vi "Actor Core.vi"(8 "error in":errorcluster, 11 "Nested in":refnum<class "Serial Devices.lvclass">) -> (0 "error out":errorcluster, 3 "Actor out":refnum<class "Actor.lvclass">)   [LabVIEW 2019, in "Serial Devices.lvlib" / "Serial Devices.lvclass"]
doc: "(<B>Filename</B>: Actor Framework.lvlib:Actor.lvclass:Actor Core.vi)\n\nReceives messages to the actor, reacts to them, and initiates any error handling that may shut the actor down.\n\nDescendant classes may override this VI to append parallel tasks for the actor to complete while it handles messages. Overrides use the Call Parent Method node."
uses:
  Serial Devices.lvclass
  <vilib>/ActorFramework/Actor/Actor.lvclass
  <vilib>/ActorFramework/Stop Msg/Stop Msg.lvclass
  Serial Devices Messages/AD Msg/AD Msg.lvclass
  C:/Program Files (x86)/National Instruments/LabVIEW 2019/vi.lib/ActorFramework/Actor/Actor.lvclass
panel:
  in  "Mandar Comando":bool
  in  "Pin":u8
  in  "Valor":u8
  in  "Puerto":u8
  in  "Canal":u8
  in  "Comandos":string(combo)="AD"
  out "Datos":string
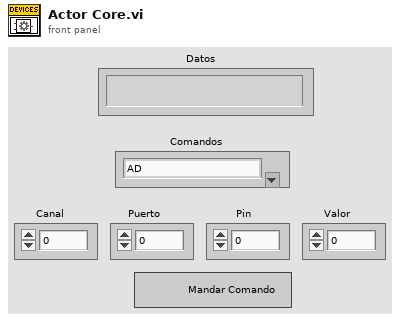
[diagram p1: front panel]
types:
  T1 = cluster{"Stop":refnum<user-event>, "Datos":refnum<user-event>}
  T2 = enum8{"Enabled", "Disabled", "Disabled and Grayed Out"}
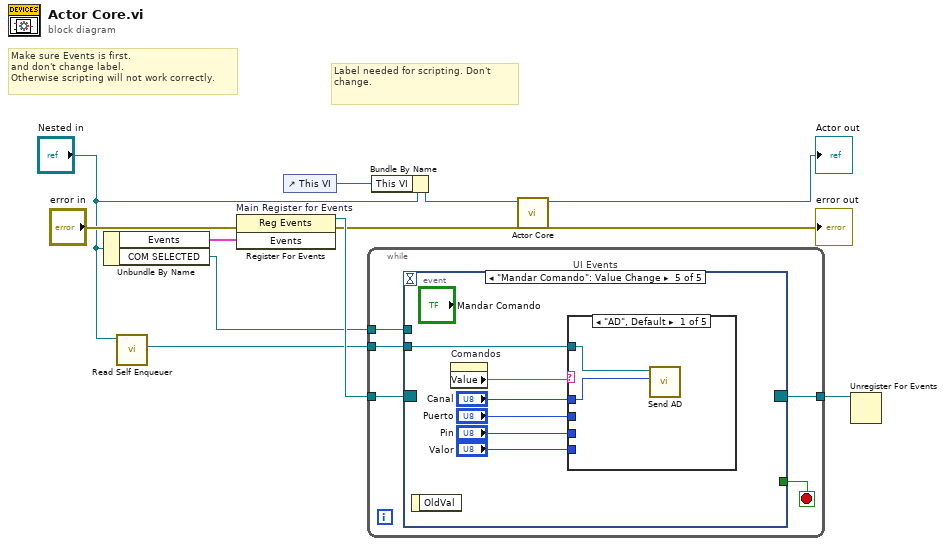
[diagram p0: block diagram]
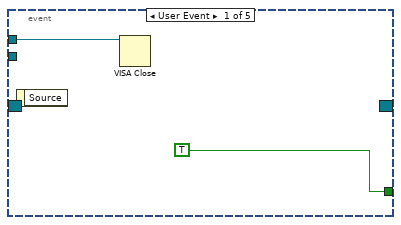
[diagram p2: hidden frame]
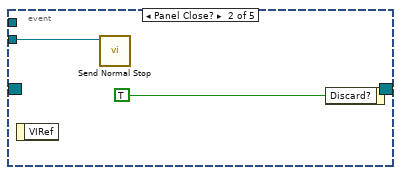
[diagram p3: hidden frame]
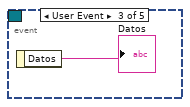
[diagram p4: hidden frame]
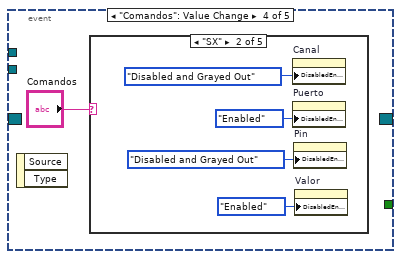
[diagram p5: hidden frame]
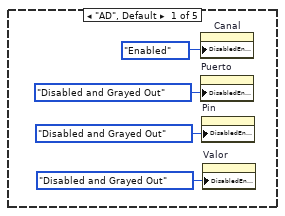
[diagram p6: hidden frame]
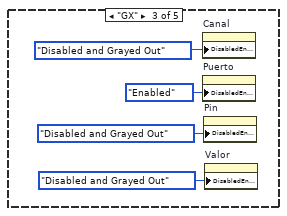
[diagram p7: hidden frame]
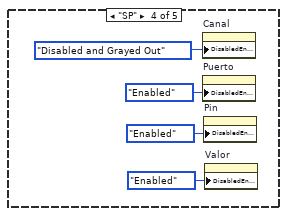
[diagram p8: hidden frame]
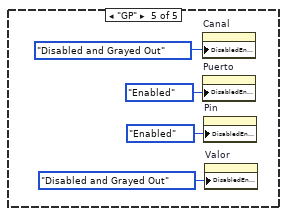
[diagram p9: hidden frame]
diagram:
  # "Label needed for scripting. Don't change."
  # "Make sure Events is first.\nand don't change label.\nOtherwise scripting will not work correctly."
  n1 = Unbundle By Name("Nested in") -> ("Events"=w9:T1, "COM SELECTED"=w1:refnum<visa-resource-name>)
  n2 = call <vilib>:"Read Self Enqueuer.vi"("Actor"="Nested in") -> ("Self Enqueuer"=w7:refnum<class "Message Enqueuer.lvclass">)  [unwired: 10 in]
  n3 = register-events "Main Register for Events"(error in="error in", w9) -> (reference out=w10:refnum<event-registration>, error out=w5:errorcluster)  [unwired: 1 in]
  n4 = control-ref of="This VI"() -> (w3:refnum<vi>)
  n5 = while {
    tunnel: w10 -> [w17]
    tunnel: [w15] -> w8
    tunnel: w7 -> [w14]
    tunnel: w1 -> [w13]
    stop <- w16 stop-if-true
    n6 = event "UI Events" shown="[4] \"Mandar Comando\": Value Change" {
      selector: w17 -> [_ _ _ _ _]
      dyn-events: [_ _ _ _ _] -> w15
      timeout: _ -> [_ _ _ _ _]
      tunnel: [TRUE _ _ _ _] -> w16
      tunnel: w14 -> [_ w20 _ _ w44]
      tunnel: w13 -> [w18 _ _ _ _]
      event User Event {
        n7 = event-data() -> ()  [unwired: 1 in, 1 out]
        n8 = VISA Close(VISA resource name=w18) -> ()  [unwired: 1 in, 1 out]
      }
      event Panel Close? {
        n9 = event-data() -> ()  [unwired: 1 in, 1 out]
        n10 = call <vilib>:"Send Normal Stop.vi"("Message Enqueuer"=w20) -> ()  [unwired: 10 in, 1 out]
        n11 = event-data("Discard?"=TRUE) -> ()  [unwired: 1 in, 1 out]
      }
      event User Event {
        n12 = event-data() -> ("Datos"=→"Datos":string)  [unwired: 1 in]
      }
      event "Comandos": Value Change {
        n13 = event-data() -> ()  [unwired: 1 in, 2 out]
        n14 = case shown="\"SX\"" "Comandos" {
          frame "AD", Default {
            n15 = property on="Canal" class="DigNum (strict)"("DisabledEnum"=T2."Enabled" ("Disabled")) -> ()  [unwired: 2 in, 2 out]
            n16 = property on="Puerto" class="DigNum (strict)"("DisabledEnum"=T2."Disabled and Grayed Out" ("Disabled")) -> ()  [unwired: 2 in, 2 out]
            n17 = property on="Pin" class="DigNum (strict)"("DisabledEnum"=T2."Disabled and Grayed Out" ("Disabled")) -> ()  [unwired: 2 in, 2 out]
            n18 = property on="Valor" class="DigNum (strict)"("DisabledEnum"=T2."Disabled and Grayed Out" ("Disabled")) -> ()  [unwired: 2 in, 2 out]
          }
          frame "SX" {
            n19 = property on="Canal" class="DigNum (strict)"("DisabledEnum"=T2."Disabled and Grayed Out" ("Disabled")) -> ()  [unwired: 2 in, 2 out]
            n20 = property on="Puerto" class="DigNum (strict)"("DisabledEnum"=T2."Enabled" ("Disabled")) -> ()  [unwired: 2 in, 2 out]
            n21 = property on="Pin" class="DigNum (strict)"("DisabledEnum"=T2."Disabled and Grayed Out" ("Disabled")) -> ()  [unwired: 2 in, 2 out]
            n22 = property on="Valor" class="DigNum (strict)"("DisabledEnum"=T2."Enabled" ("Disabled")) -> ()  [unwired: 2 in, 2 out]
          }
          frame "GX" {
            n23 = property on="Canal" class="DigNum (strict)"("DisabledEnum"=T2."Disabled and Grayed Out" ("Disabled")) -> ()  [unwired: 2 in, 2 out]
            n24 = property on="Puerto" class="DigNum (strict)"("DisabledEnum"=T2."Enabled" ("Disabled")) -> ()  [unwired: 2 in, 2 out]
            n25 = property on="Pin" class="DigNum (strict)"("DisabledEnum"=T2."Disabled and Grayed Out" ("Disabled")) -> ()  [unwired: 2 in, 2 out]
            n26 = property on="Valor" class="DigNum (strict)"("DisabledEnum"=T2."Disabled and Grayed Out" ("Disabled")) -> ()  [unwired: 2 in, 2 out]
          }
          frame "SP" {
            n27 = property on="Canal" class="DigNum (strict)"("DisabledEnum"=T2."Disabled and Grayed Out" ("Disabled")) -> ()  [unwired: 2 in, 2 out]
            n28 = property on="Puerto" class="DigNum (strict)"("DisabledEnum"=T2."Enabled" ("Disabled")) -> ()  [unwired: 2 in, 2 out]
            n29 = property on="Pin" class="DigNum (strict)"("DisabledEnum"=T2."Enabled" ("Disabled")) -> ()  [unwired: 2 in, 2 out]
            n30 = property on="Valor" class="DigNum (strict)"("DisabledEnum"=T2."Enabled" ("Disabled")) -> ()  [unwired: 2 in, 2 out]
          }
          frame "GP" {
            n31 = property on="Canal" class="DigNum (strict)"("DisabledEnum"=T2."Disabled and Grayed Out" ("Disabled")) -> ()  [unwired: 2 in, 2 out]
            n32 = property on="Puerto" class="DigNum (strict)"("DisabledEnum"=T2."Enabled" ("Disabled")) -> ()  [unwired: 2 in, 2 out]
            n33 = property on="Pin" class="DigNum (strict)"("DisabledEnum"=T2."Enabled" ("Disabled")) -> ()  [unwired: 2 in, 2 out]
            n34 = property on="Valor" class="DigNum (strict)"("DisabledEnum"=T2."Disabled and Grayed Out" ("Disabled")) -> ()  [unwired: 2 in, 2 out]
          }
        }
      }
      event "Mandar Comando": Value Change {
        n35 = event-data() -> ()  [unwired: 1 in, 1 out]
        n36 = property on="Comandos" class="CmbBox"() -> ("Value"=w49:string)  [unwired: 2 in, 2 out]
        n37 = case shown="\"AD\", Default" w49 {
          tunnel: "Canal" -> [w50 _ _ _ _]
          tunnel: "Puerto" -> [_ _ _ _ _]
          tunnel: "Pin" -> [_ _ _ _ _]
          tunnel: "Valor" -> [_ _ _ _ _]
          tunnel: w44 -> [w51 _ _ _ _]
          frame "AD", Default {
            n38 = call "Send AD.vi"("Canal"=w50, "Message Enqueuer"=w51) -> ()  [unwired: 8 in, 2 out]
          }
          frame "SX" {
          }
          frame "GX" {
          }
          frame "SP" {
          }
          frame "GP" {
          }
        }
      }
    }
  }
  n39 = Bundle By Name(cluster="Nested in", "This VI"=w3) -> (w4:refnum<class "Serial Devices.lvclass">)
  n40 = call-parent "Actor Core.vi"("error in"=w5, "Actor in"=w4) -> ("error out"=→"error out":errorcluster, "Actor out"=→"Actor out":refnum<class "Actor.lvclass">)  [unwired: 8 in]
  n41 = Unregister For Events(event registration refnum=w8) -> ()  [unwired: 1 in, 1 out]
